vi "thermal camera.vi"() -> ()   [LabVIEW 2024]
uses:
  <vilib>/userDefined/High Color/IMAQdx.ctl
  <vilib>/vision/driver/NI_Vision_Acquisition_Software.lvlib
panel:
  out "Image":T1(plugin-control)
  in  "stop":bool
  in  "Session In":T2
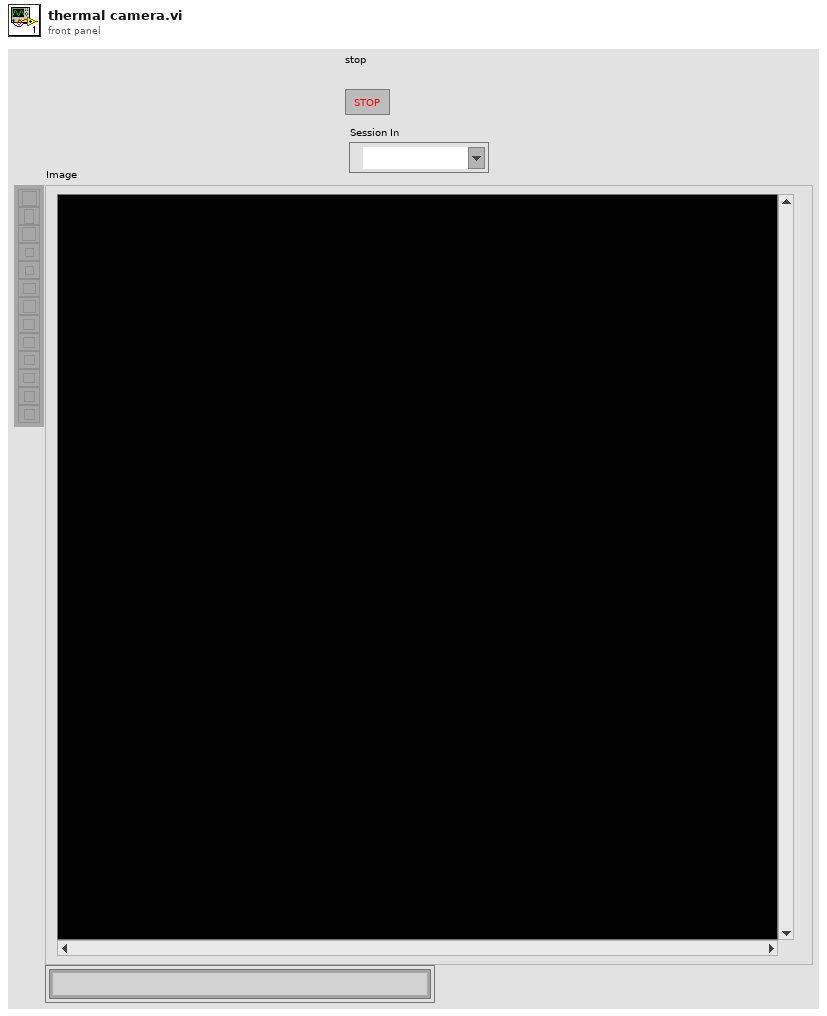
[diagram p1: front panel]
types:
  T1 = typedef "IMAQ Image.ctl" = refnum<image>
  T2 = typedef "IMAQdx.ctl" = refnum<k21>
  T3 = typedef "Image Type" = u32
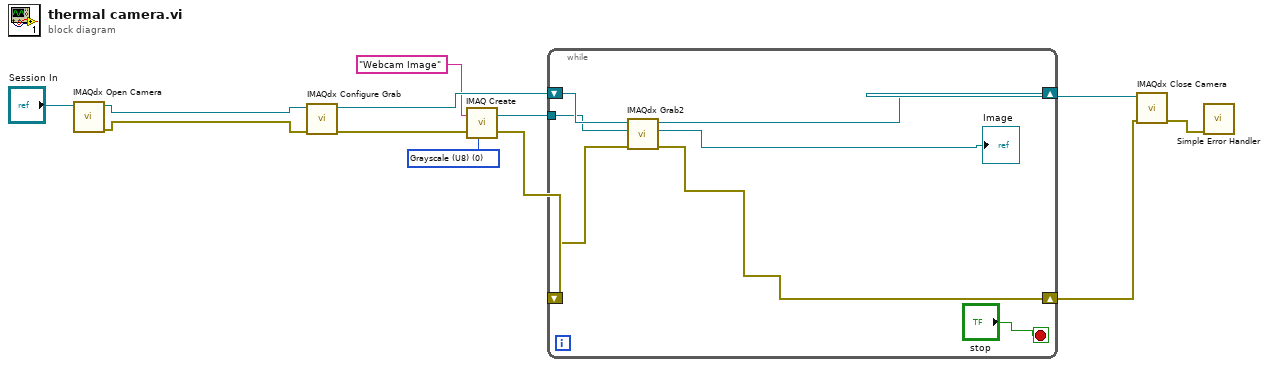
[diagram p0: block diagram]
diagram:
  w3 = T3 0 items=["Grayscale (U8)", "Grayscale (I16)", "Grayscale (SGL)", "Complex (CSG)", "RGB (U32)", "HSL (U32)", "RGB (U64)", "Grayscale (U16)"] ("Image Type")
  n1 = call <vilib>:"IMAQdx Open Camera.vi"("Session In"="Session In") -> ("error out"=w2:errorcluster, "Session Out"=w1:T2)  [unwired: 9 in]
  n2 = call <vilib>:"IMAQdx Configure Grab.vi"("error in"=w2, "Session In"=w1) -> ("error out"=w5:errorcluster, "Session Out"=w11:T2)  [unwired: 8 in]
  n3 = call "IMAQ Create"("Image Name"="Webcam Image", "Image Type"=w3, "error in (no error)"=w5) -> ("New Image"=w7:T1, "error out"=w4:errorcluster)  [unwired: 2 in]
  n4 = while {
    shift-right: [w18] -> w10
    shift-left: w11 -> [w19]
    shift-right: [w13] -> w9
    shift-left: w4 -> [w17]
    tunnel: w7 -> [w15]
    stop <- "stop" stop-if-true
    n5 = call <vilib>:"IMAQdx Grab2.vi"("error in"=w17, "Image In"=w15, "Session In"=w19) -> ("error out"=w13:errorcluster, "Image Out"=→"Image":T1, "Session Out"=w18:T2)  [unwired: 5 in, 1 out]
  }
  n6 = call <vilib>:"IMAQdx Close Camera.vi"("error in"=w9, "Session In"=w10) -> ("error out"=w6:errorcluster)  [unwired: 9 in]
  n7 = call <vilib>:"Simple Error Handler.vi"("error in (no error)"=w6) -> ()  [unwired: 4 in, 5 out]
